vi "pwm.vi"(1 "Frequency (Hz)":sgl, 2 "Duty Cycle (%)":sgl, 3 "FPGA I/O In":refnum<k21>="ConnectorB/DIO1") -> ()   [LabVIEW 2019]
uses:
  <vilib>/rvi/eio/common/nirviEmuTemplateMethod_errors.vi
  <vilib>/eio/EIONode/EIONode.xnode
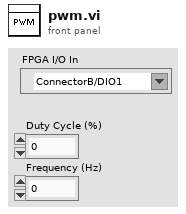
[diagram p1: front panel]
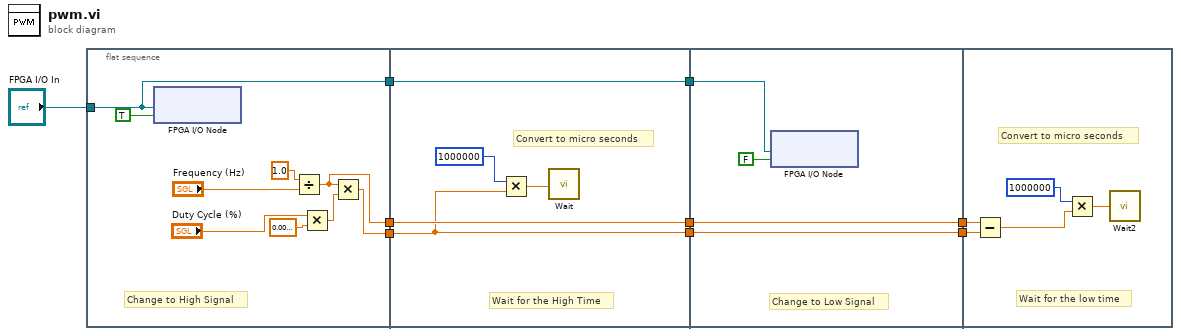
[diagram p0: block diagram]
diagram:
  n1 = flat-sequence {
    tunnel: [w12] -> w9
    tunnel: [w17] -> w8
    tunnel: "FPGA I/O In" -> [w10]
    tunnel: [w10] -> w7
    tunnel: w9 -> [w23]
    tunnel: [w23] -> w6
    tunnel: w8 -> [w21]
    tunnel: [w21] -> w5
    tunnel: w7 -> [w19]
    tunnel: [w19] -> w4
    tunnel: w6 -> [w26]
    tunnel: w5 -> [w27]
    tunnel: [w27] -> w3
    tunnel: [w26] -> w2
    tunnel: w4 -> [w24]
    tunnel: w3 -> [w32]
    tunnel: w2 -> [w31]
    frame #0 {
      # "Change to High Signal"
      n2 = xnode "FPGA I/O Node"("I/O Item"=TRUE, "FPGA I/O In"=w10) -> ()  [unwired: 1 out]
      n3 = Divide(x=sgl 1.0 ("Frequency (Hz)) 2"), y="Frequency (Hz)") -> (x/y=w12:sgl)
      n4 = Multiply(x="Duty Cycle (%)", y=sgl 0.01) -> (x*y=w15:sgl)
      n5 = Multiply(x=w12, y=w15) -> (x*y=w17:sgl)
    }
    frame #1 {
      # "Wait for the High Time"
      # "Convert to micro seconds"
      n6 = Multiply(x=u32 1000000, y=w21) -> (x*y=w20:sgl)
      n7 = call "Wait"("Count(uSec)"=w20) -> ()  [unwired: 1 out]
    }
    frame #2 {
      # "Change to Low Signal"
      n8 = xnode "FPGA I/O Node"("I/O Item"=FALSE, "FPGA I/O In"=w24) -> ()  [unwired: 1 out]
    }
    frame #3 {
      # "Convert to micro seconds"
      # "Wait for the low time"
      n9 = Subtract(x=w31, y=w32) -> (x-y=w28:sgl)
      n10 = Multiply(x=u32 1000000, y=w28) -> (x*y=w29:sgl)
      n11 = call "Wait2"("Count(uSec)"=w29) -> ()  [unwired: 1 out]
    }
  }
